vi "Get TreeItem Children Indices.vi"(10 "TreeItem Index":i32, 11 "TreeItems":T1[](array[typedef])) -> (2 "TreeItem index indent":i32, 3 "Child indices (incrementing)":i32[](array[numeric]))   [LabVIEW 2020, in "BetterDragAndDrop.lvlib" / "BetterTreeHandle.lvclass"]
uses:
  BetterTreeHandle/BetterTreeHandle.lvclass
  TreeItem.ctl
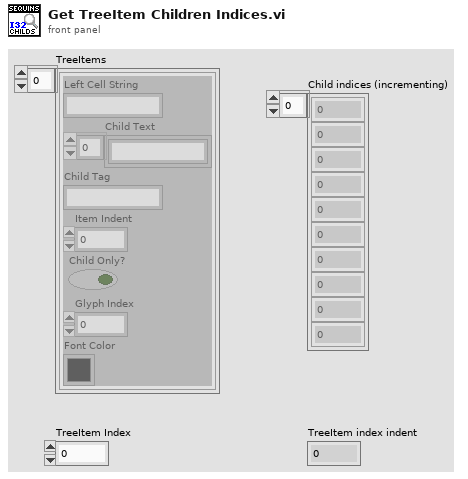
[diagram p1: front panel]
types:
  T1 = typedef "BetterDragAndDrop.lvlib/BetterTreeHandle.lvclass/TreeItem.ctl" = cluster{"Left Cell String":string, "Child Text":string[], "Child Tag":string, "Item Indent":i32, "Child Only?":bool, "Glyph Index":i32, "Font Color":u32}
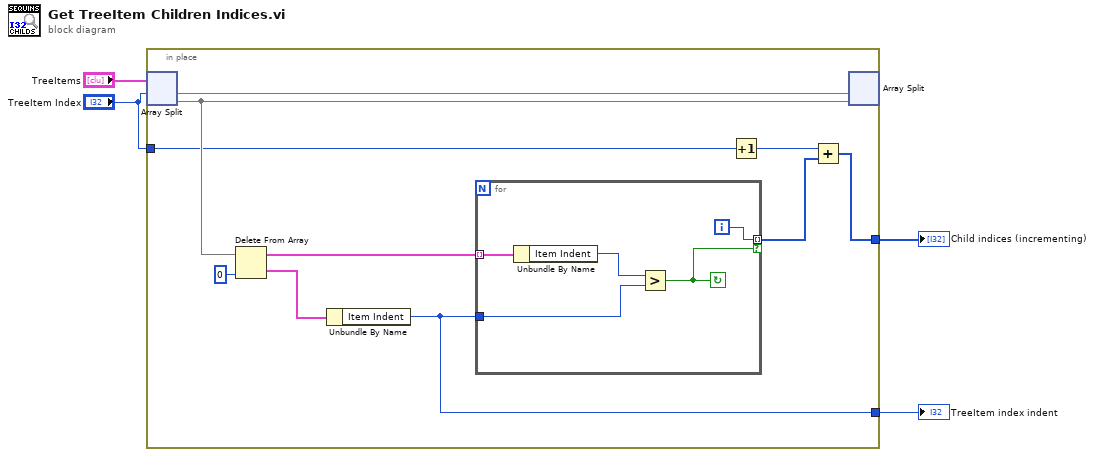
[diagram p0: block diagram]
diagram:
  n1 = in-place {
    in-place-border: [w14] -> w3
    in-place-border: [w9] -> w2
    in-place-border: "TreeItem Index" -> [w6]
    n2 = in-place-split #1("TreeItems", "TreeItem Index") -> (w10:T1[], w7:T1[])
    n3 = Delete From Array(array=w7, index=0) -> (deleted portion=w12:T1, array with subset deleted=w11:T1[])  [unwired: 1 in]
    n4 = Unbundle By Name(w12) -> ("Item Indent"=w9:i32)
    n5 = for {
      tunnel: w11 -> [w19] mode=indexing
      tunnel: [w18] -> w8 mode=indexing if=w15
      tunnel: w9 -> [w16]
      i -> [w18]
      stop <- w15 continue-if-true
      n6 = Unbundle By Name(w19) -> ("Item Indent"=w17:i32)
      n7 = Greater?(x=w17, y=w16) -> (0:w15:bool)
    }
    n8 = Increment(x=w6) -> (x+1=w5:i32)
    n9 = Add(x=w5, y=w8) -> (x+y=w14:i32[])
    n10 = in-place-split #1(w10, w7) -> ()  [unwired: 2 out]
  }
  "Child indices (incrementing)" <- w3
  "TreeItem index indent" <- w2
